vi "VariableInjector.vi"(10 "Variables":T1(array[cluster]), 11 "Expression":string) -> (2 "Result":string)   [LabVIEW 2012]
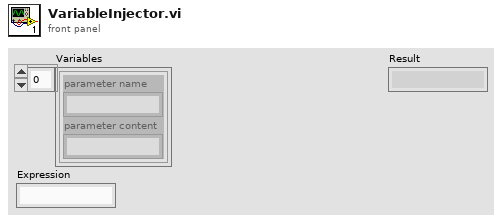
[diagram p1: front panel]
types:
  T1 = cluster{"parameter name":string, "parameter content":string}[]
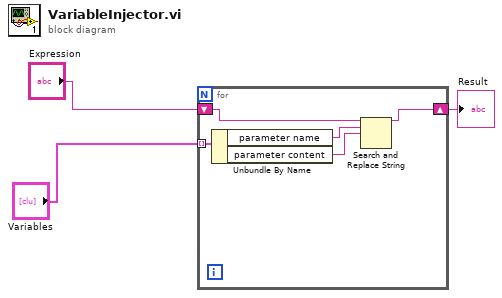
[diagram p0: block diagram]
diagram:
  n1 = for {
    tunnel: "Variables" -> [w8] mode=indexing
    shift-right: [w4] -> w1
    shift-left: "Expression" -> [w5]
    n2 = Unbundle By Name(w8) -> ("parameter name"=w6:string, "parameter content"=w7:string)
    n3 = Search and Replace String(input string=w5, search string=w6, replace string=w7) -> (result string=w4:string)  [unwired: 5 in, 3 out]
  }
  "Result" <- w1
